vi "TBM.ScrollBarsOFF.vi"(8 "error in (no error)":errorcluster, 11 "VI in":refnum<vi>) -> (0 "error out":errorcluster, 3 "VI out":refnum<vi>)   [LabVIEW 2013, in "ToolbarMenu.lvlib"]
uses:
  ToolbarMenu.lvlib
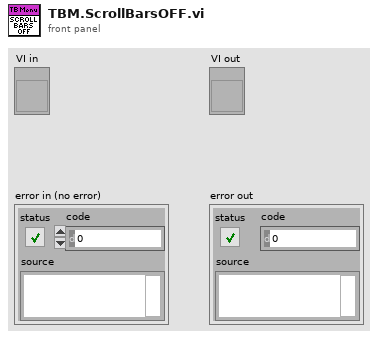
[diagram p1: front panel]
types:
  T1 = enum16{"Always On", "Always Off", "Off While Running"}
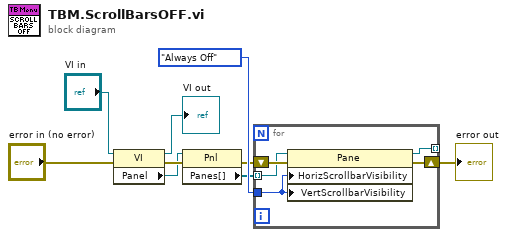
[diagram p0: block diagram]
diagram:
  n1 = property class="VI"(reference="VI in", error in="error in (no error)") -> (reference out=→"VI out":refnum<vi>, error out=w2:errorcluster, "Panel"=w1:refnum<vi>)
  n2 = property class="Pnl"(reference=w1, error in=w2) -> (error out=w3:errorcluster, "Panes[]"=w4:refnum<vi>[])  [unwired: 1 out]
  n3 = for {
    shift-right: [w13] -> w7
    shift-left: w3 -> [w14]
    tunnel: w4 -> [w12] mode=indexing
    tunnel: [w11] -> _ mode=indexing
    tunnel: T1."Always Off" ("All Scrollbar Visibility") -> [w10]
    n4 = property class="Pane"(reference=w12, error in=w14, "HorizScrollbarVisibility"=w10, "VertScrollbarVisibility"=w10) -> (reference out=w11:refnum<vi>, error out=w13:errorcluster)
  }
  "error out" <- w7
